vi "ROI_Picture_size.vi"(8 "Input Cluster":T6, 11 "Pixel":T7) -> (0 "output cluster":T6)   [LabVIEW 2009]
uses:
  atmcd32d.llb/AcquisitionMode_mode typedef.ctl
  atmcd32d.llb/ReadMode_mode typedef.ctl
  atmcd32d.llb/TriggerMode_mode typedef.ctl
  atmcd32d.llb/Shutter_type typedef.ctl
  atmcd32d.llb/Shutter_mode typedef.ctl
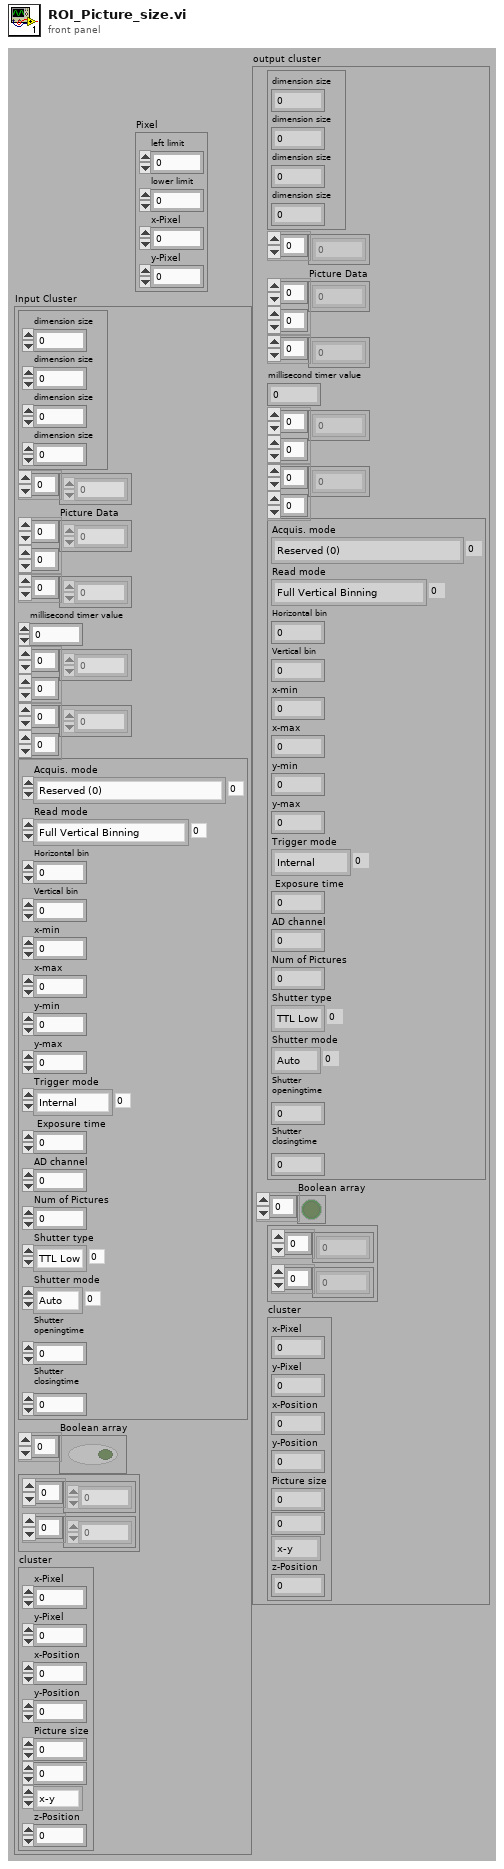
[diagram p1: front panel]
types:
  T1 = typedef "AcquisitionMode_mode typedef.ctl" = enum16{"Reserved (0)", "Single Scan", "Accumulate", "Kinetics", "Fast Kinetics", "Run Till Abort", "Reserved (6)", "Reserved (7)", "Reserved (8)", "Time Delayed Integration"}
  T2 = typedef "ReadMode_mode typedef.ctl" = enum16{"Full Vertical Binning", "Multi-Track", "Random-Track", "Single-Track", "Image"}
  T3 = typedef "TriggerMode_mode typedef.ctl" = enum16{"Internal", "External", "N/A (2)", "N/A (3)", "N/A (4)", "N/A (5)", "External Start"}
  T4 = typedef "Shutter_type typedef.ctl" = enum16{"TTL Low", "TTL High"}
  T5 = typedef "Shutter_mode typedef.ctl" = enum16{"Auto", "Open", "Close"}
  T6 = cluster{cluster{"dimension size":i32, "dimension size":i32, "dimension size":i32, "dimension size":i32}, i32[], "Picture Data":dbl[][], u32[], "millisecond timer value":u32, dbl[][], i32[][], cluster{"Acquis. mode":T1, "Read mode":T2, "Horizontal bin":i32, "Vertical bin":i32, "x-min":i32, "x-max":i32, "y-min":i32, "y-max":i32, "Trigger mode":T3, " Exposure time":sgl, "AD channel":i32, "Num of Pictures":i32, "Shutter type":T4, "Shutter mode":T5, "Shutter\nopeningtime":i32, "Shutter\nclosingtime":i32}, "Boolean array":bool[], cluster{dbl[], dbl[]}, "cluster":cluster{"x-Pixel":u16, "y-Pixel":u16, "x-Position":dbl, "y-Position":dbl, "Picture size":dbl, dbl, enum32{"x-y", "x-z", "y-z"}, "z-Position":dbl}}
  T7 = cluster{"left limit":i32, "lower limit":i32, "x-Pixel":i32, "y-Pixel":i32}
  T8 = cluster{"x-Pixel":u16, "y-Pixel":u16, "x-Position":dbl, "y-Position":dbl, "Picture size":dbl, dbl, enum32{"x-y", "x-z", "y-z"}, "z-Position":dbl}
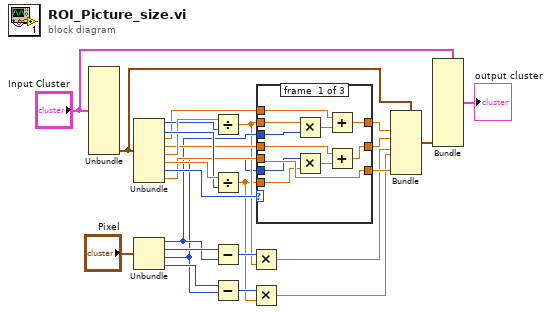
[diagram p0: block diagram]
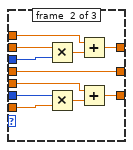
[diagram p2: hidden frame]
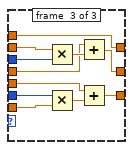
[diagram p3: hidden frame]
diagram:
  n1 = Unbundle("Input Cluster") -> ("cluster"=w17:T8)  [unwired: 10 out]
  n2 = Unbundle(w17) -> ("x-Pixel"=w22:u16, "y-Pixel"=w24:u16, "x-Position"=w20:dbl, "y-Position"=w19:dbl, "Picture size"=w23:dbl, w25:dbl, w21:enum32{"x-y", "x-z", "y-z"}, "z-Position"=w18:dbl)
  n3 = Unbundle("Pixel") -> ("left limit"=w9:i32, "lower limit"=w10:i32, "x-Pixel"=w2:i32, "y-Pixel"=w3:i32)
  n4 = Divide(x=w23, y=w22) -> (x/y=w7:dbl)
  n5 = Divide(x=w25, y=w24) -> (x/y=w4:dbl)
  n6 = Subtract(x=w10, y=w9) -> (x-y=w8:i32)
  n7 = Subtract(x=w3, y=w2) -> (x-y=w5:i32)
  n8 = Multiply(x=w8, y=w7) -> (x*y=w6:dbl)
  n9 = Multiply(x=w5, y=w4) -> (x*y=w1:dbl)
  n10 = case shown="\"x-z\"" w21 {
    tunnel: w20 -> [w33 w42 w49]
    tunnel: w19 -> [w28 w38 w53]
    tunnel: w18 -> [w37 w40 w51]
    tunnel: [w31 w41 w49] -> w16
    tunnel: [w29 w38 w52] -> w15
    tunnel: [w37 w39 w50] -> w14
    tunnel: w7 -> [w36 w43 w54]
    tunnel: w4 -> [w34 w44 w55]
    tunnel: w9 -> [w27 w45 w56]
    tunnel: w2 -> [w35 w46 w57]
    frame #0 {
      n11 = Multiply(x=w36, y=w27) -> (x*y=w32:dbl)
      n12 = Multiply(x=w35, y=w34) -> (x*y=w30:dbl)
      n13 = Add(x=w33, y=w32) -> (x+y=w31:dbl)
      n14 = Add(x=w28, y=w30) -> (x+y=w29:dbl)
    }
    frame #1 {
      n15 = Multiply(x=w43, y=w45) -> (x*y=w48:dbl)
      n16 = Multiply(x=w46, y=w44) -> (x*y=w47:dbl)
      n17 = Add(x=w42, y=w48) -> (x+y=w41:dbl)
      n18 = Add(x=w40, y=w47) -> (x+y=w39:dbl)
    }
    frame #2 {
      n19 = Multiply(x=w54, y=w56) -> (x*y=w59:dbl)
      n20 = Multiply(x=w57, y=w55) -> (x*y=w58:dbl)
      n21 = Add(x=w53, y=w59) -> (x+y=w52:dbl)
      n22 = Add(x=w51, y=w58) -> (x+y=w50:dbl)
    }
  }
  n23 = Bundle(cluster=w17, "x-Position"=w16, "y-Position"=w15, "Picture size"=w6, w1, "z-Position"=w14) -> (w12:T8)  [unwired: 3 out]
  n24 = Bundle(cluster="Input Cluster", "cluster"=w12) -> (→"output cluster":T6)  [unwired: 10 out]
